vi "IMUOrientOpen.vi"(4 "Flash Drive?":bool, 5 "Stored Cal File":string="BNO055 Cal MC P3 11-28-2015 145653", 6 "Alt Adr":bool, 7 "Calibrate?":bool, 8 "Status delay":i32=30, 9 "I2C Bus":T2=enum."I2C MXP", 10 "Placement":T7(ring)=enum."P3", 11 "Op Mode":T5(ring)=enum."NDOF") -> (0 "Bad result":bool, 1 "Fatal Result":bool, 2 "Cal Status":T3, 3 "I2CDevRef":T1={"DevStatus"={"status"=FALSE, "code"=0, "source"=""}, "Device Address"=0, "Handle"=0, "I2C Bus"=enum."Invalid"} {"Device Address" format="%.0x"})   [LabVIEW 2015]
uses:
  <vilib>/Rock Robotics/SystemInterfaces/i2clib/i2c_bus.ctl
  Setup State.ctl
  <vilib>/Rock Robotics/WPI/I2C/WPI_I2CDevRef.ctl
panel:
  out "Adr":u8 format="%02x"
  out "Fatal Result":bool
  out "Restore Cal Ct":i32
  out "Bad ct":i32
  out "SC ct":i32
  out "S":T4
  out "G":T4
  out "A":T4
  out "M":T4
  out "Bad result":bool
  out "Fusion":bool
  out "Fusion ct":i32
  out "Reset ct":i32
  out "Occupant":u8[](array[numeric]) format="%02x"
  out "Setup ct":i32
  out "Setup State":T6
  # "Manual Cal\nCalibration Status Indicator"
  # "Diagnostics"
  # "These controls/indicators are non-operational / they are here as example documentation only."
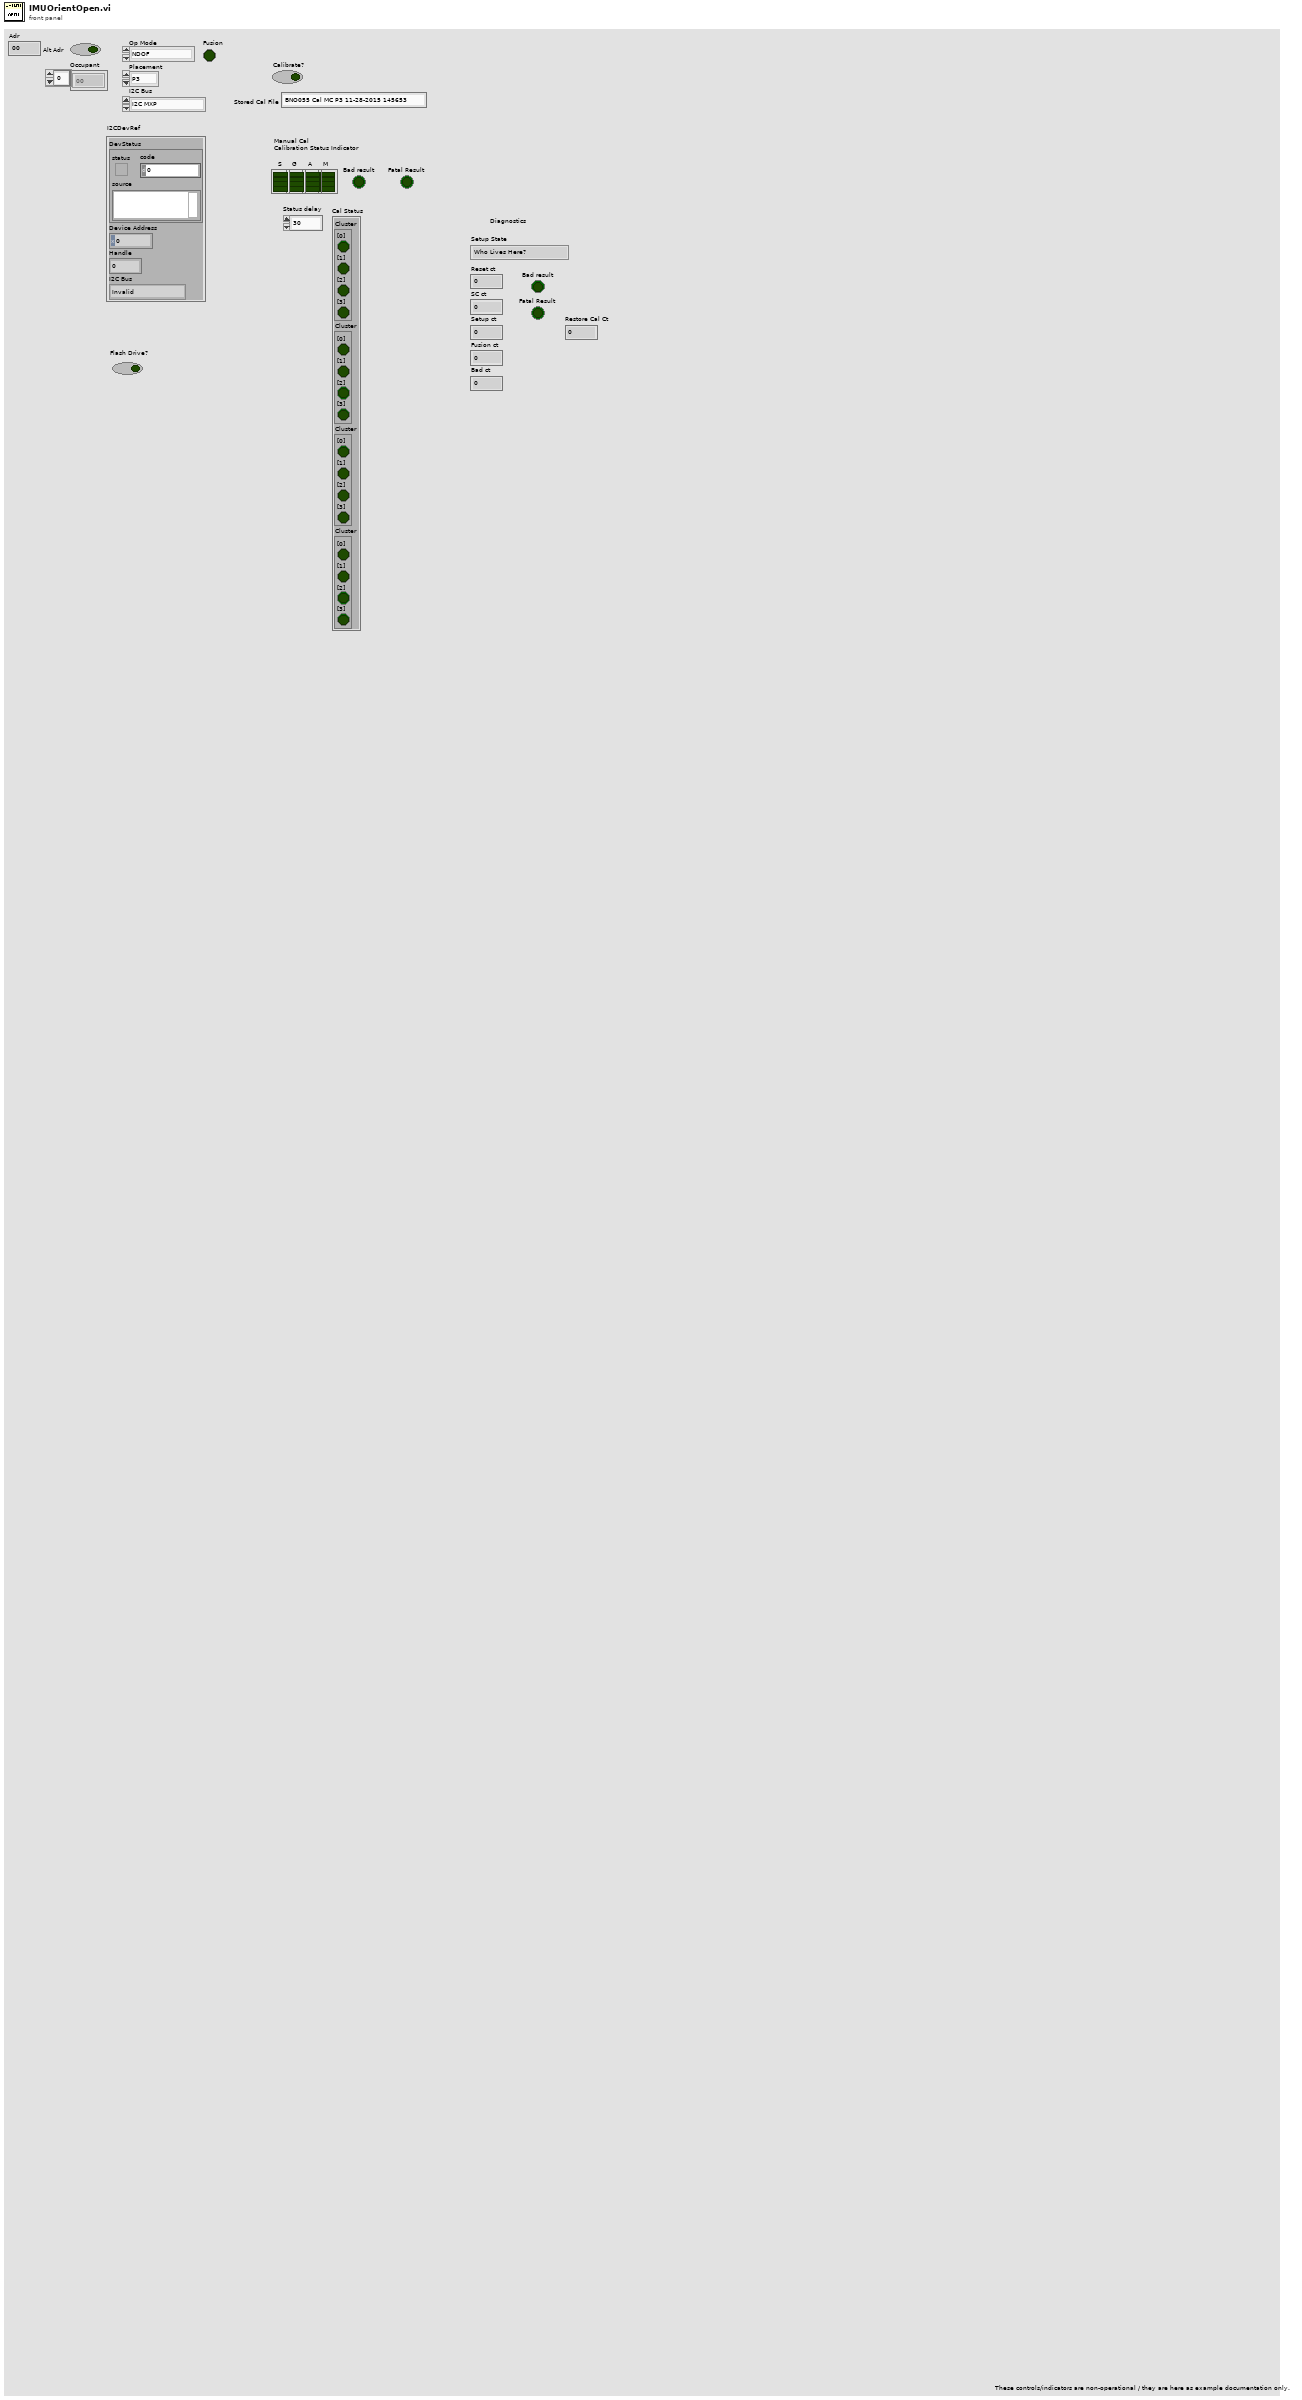
[diagram p1: front panel]
types:
  T1 = typedef "WPI_I2CDevRef.ctl" = cluster{"DevStatus":errorcluster, "Device Address":u8, "Handle":i32, "I2C Bus":T2}
  T2 = typedef "i2c_bus.ctl" = enum16{"I2C On-Board", "I2C MXP", "Invalid"}
  T3 = cluster{"Cluster":cluster{"[0]":bool, "[1]":bool, "[2]":bool, "[3]":bool}, "Cluster":cluster{"[0]":bool, "[1]":bool, "[2]":bool, "[3]":bool}, "Cluster":cluster{"[0]":bool, "[1]":bool, "[2]":bool, "[3]":bool}, "Cluster":cluster{"[0]":bool, "[1]":bool, "[2]":bool, "[3]":bool}}
  T4 = cluster{"Boolean":bool, "Boolean 2":bool, "Boolean 3":bool, "Boolean 4":bool}
  T5 = enum8{"ConfigMode", "AccOnly", "MagOnly", "GyroOnly", "AccMag", "AccGyro", "MagGyro", "AMG", "IMU", "Compass", "M4G", "NDOF_FMC_OFF", "NDOF"}
  T6 = typedef "Setup State.ctl" = enum16{"Who Lives Here?", "Config Mode", "Page 0", "Reset", "Units, Xtal, & Placement", "Fusion Mode", "Pre Calibration", "Error Check", "Manual Cal", "Save Cal", "Restore Cal", "Cal Status", "Idle"}
  T7 = enum32{"P0", "P1", "P2", "P3", "P4", "P5", "P6", "P7"}
  T8 = enum16{"open", "open or create", "create or replace", "create", "open (read-only)"}
  T9 = enum8{"ConfigMode", "AccOnly", "MagOnly", "GyroOnly", "AccMag", "AccGyro", "MagGyro", "AMG", "IMU", "Compass", "M4G", "NDOF_FMC_OFF", "NDOF"}[]
  T10 = cluster{"[0]":bool, "[1]":bool, "[2]":bool, "[3]":bool}
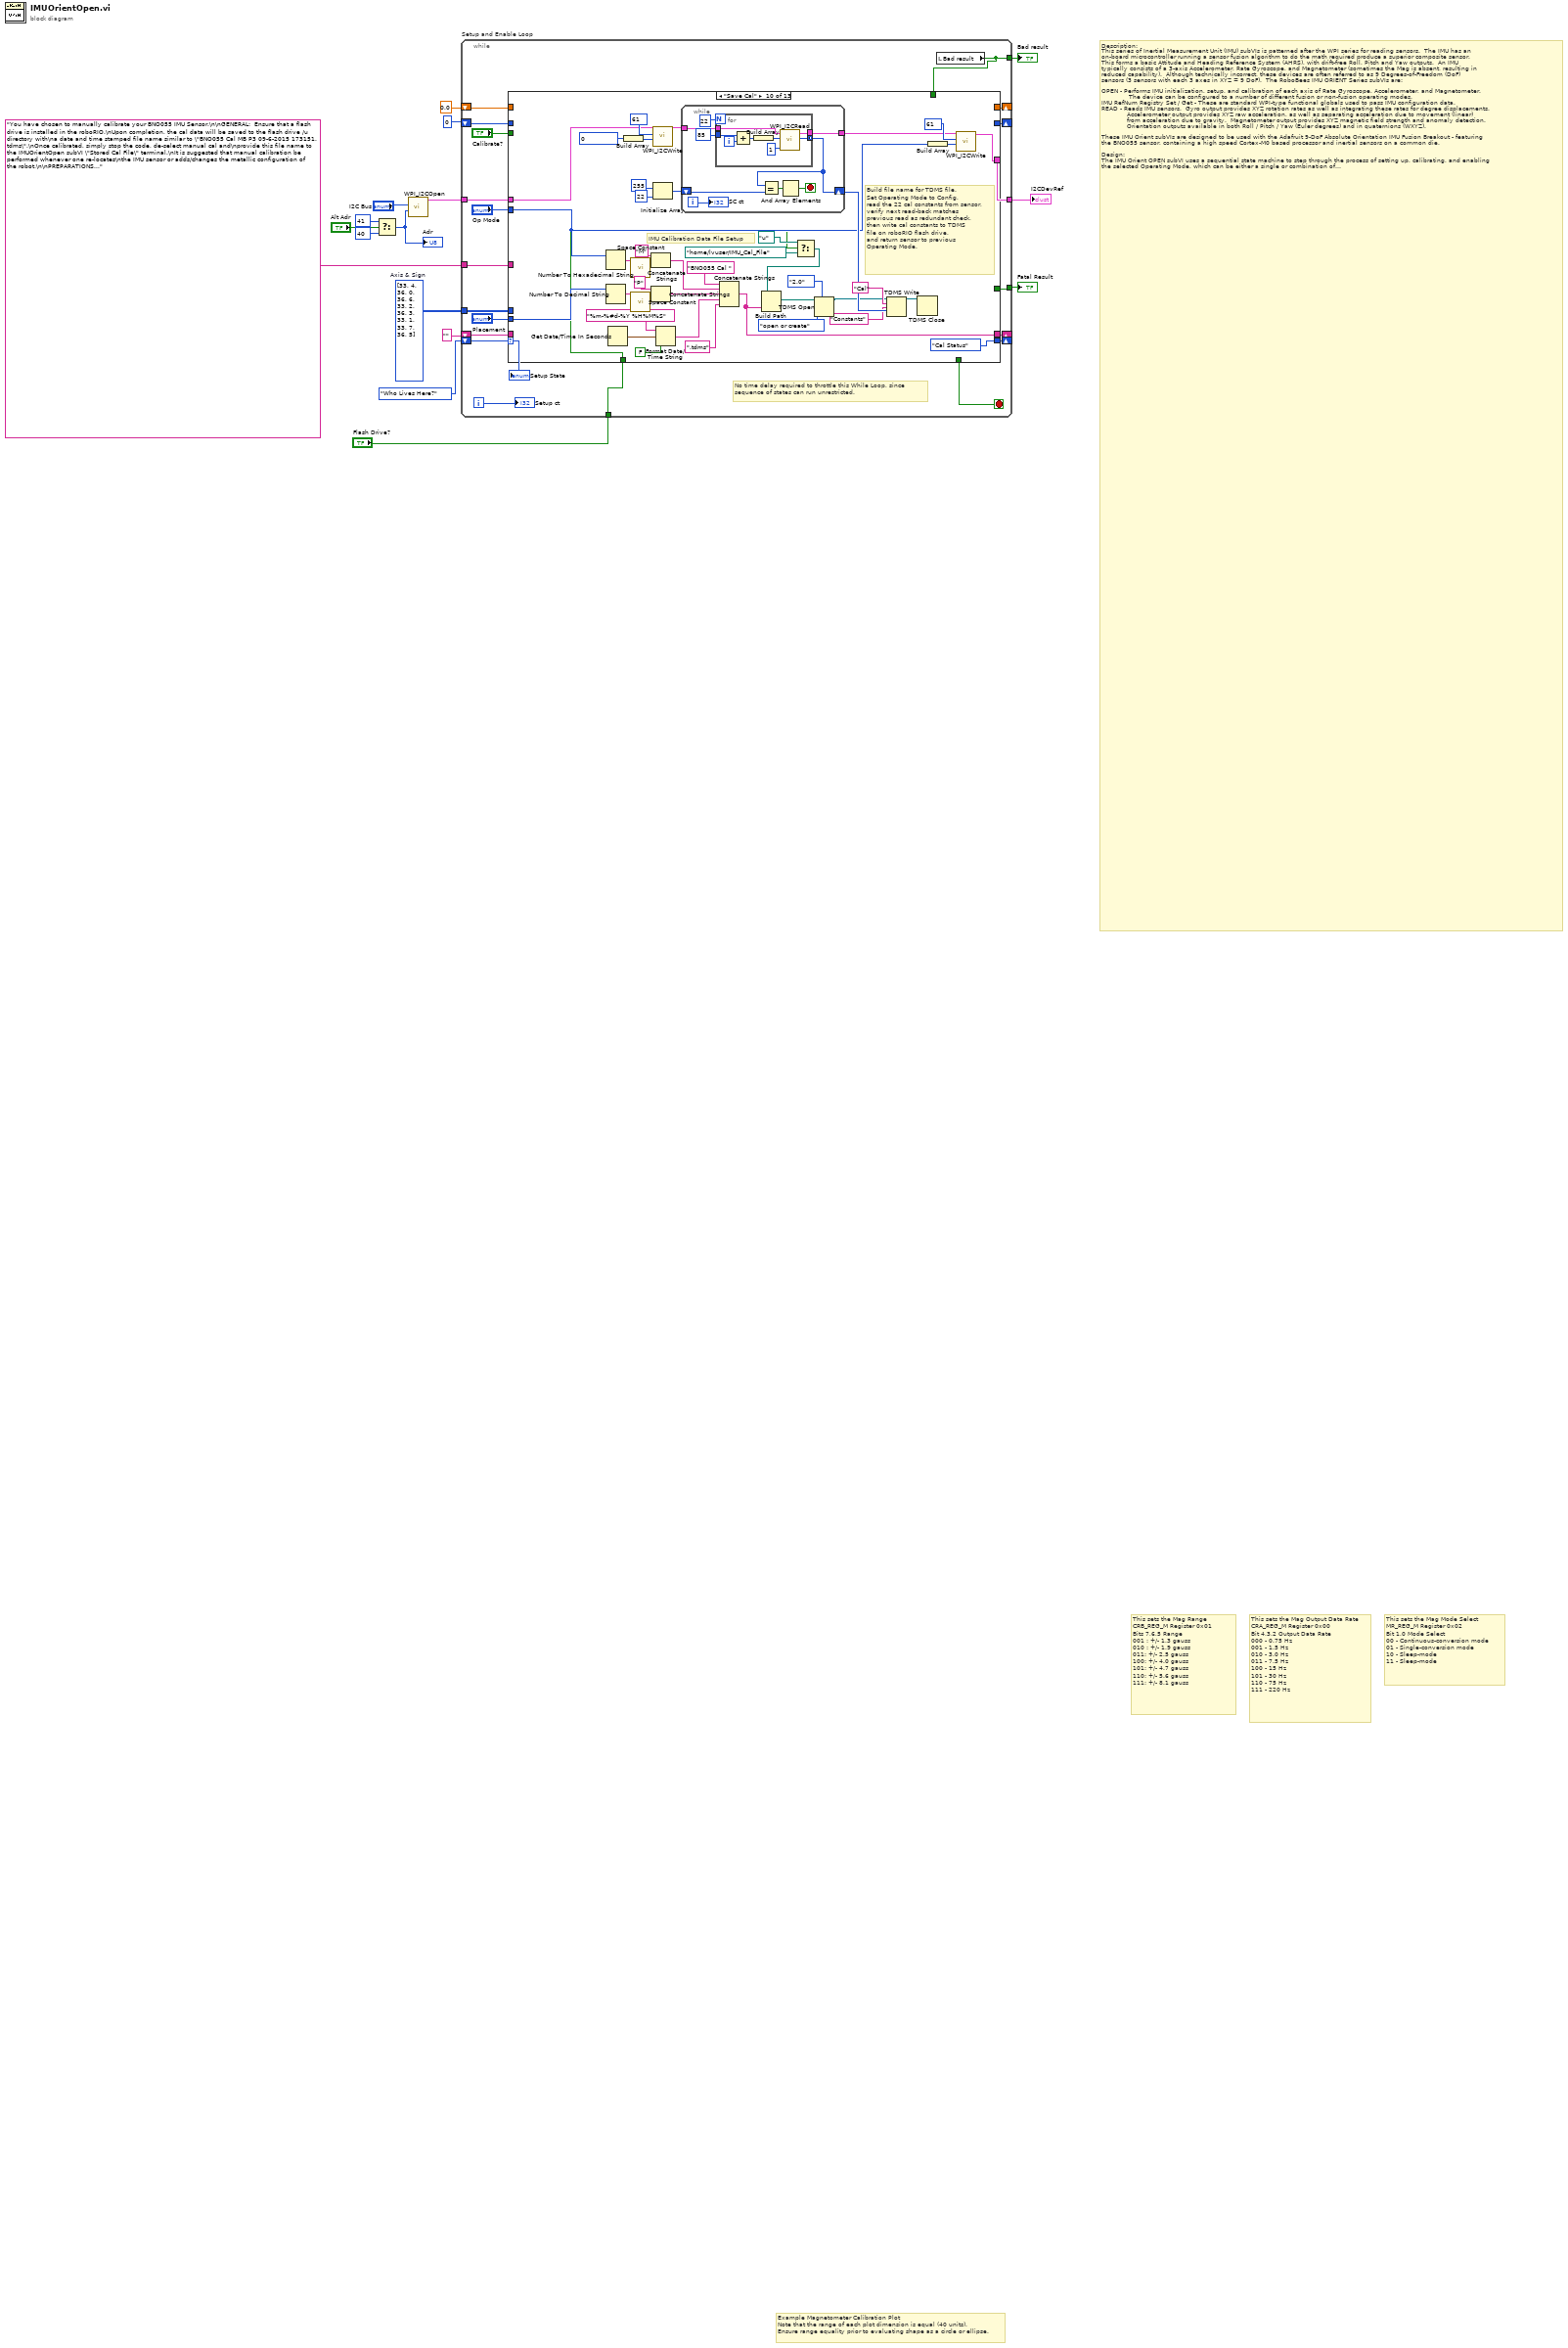
[diagram p0: block diagram]
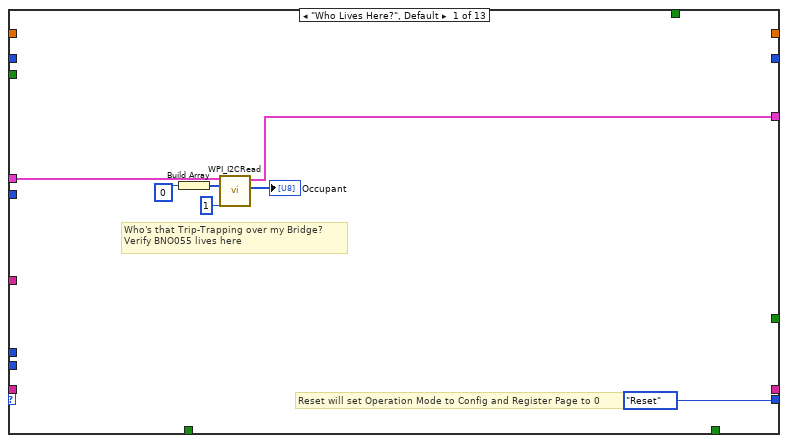
[diagram p2: hidden frame]
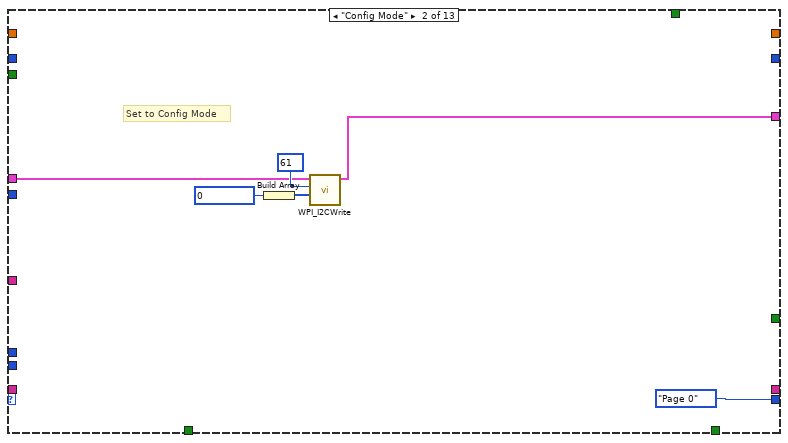
[diagram p3: hidden frame]
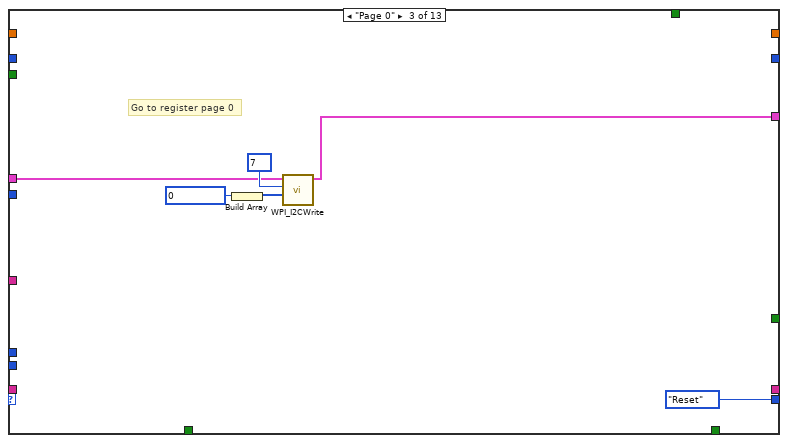
[diagram p4: hidden frame]
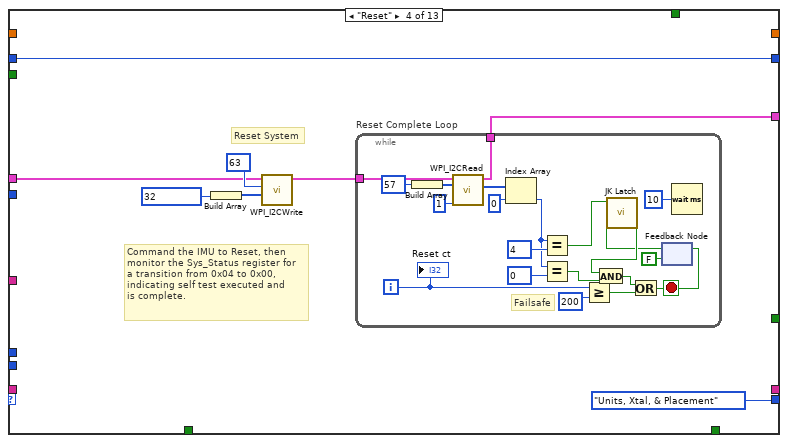
[diagram p5: hidden frame]
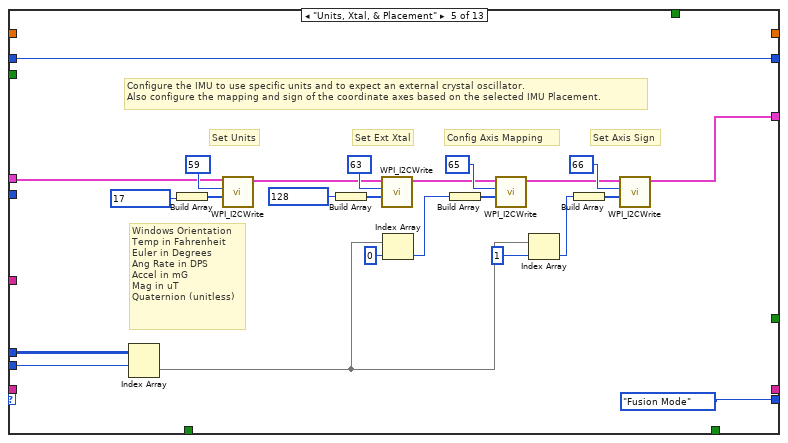
[diagram p6: hidden frame]
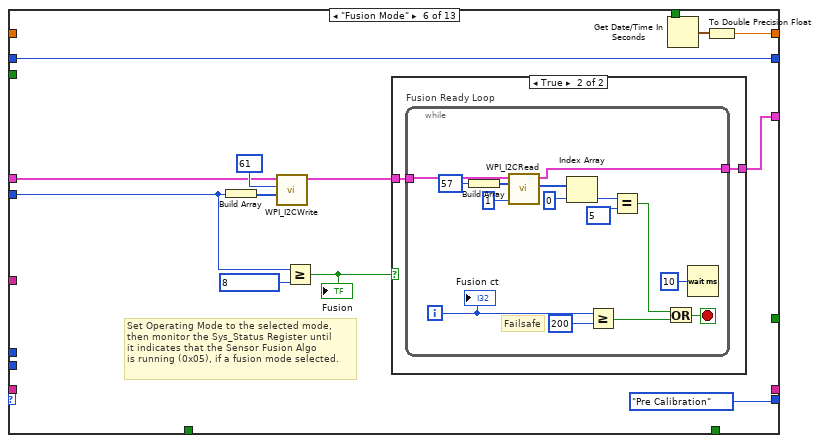
[diagram p7: hidden frame]
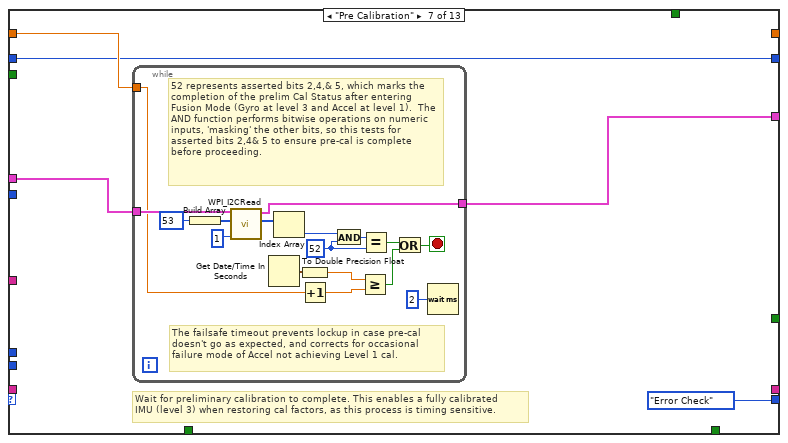
[diagram p9: hidden frame]
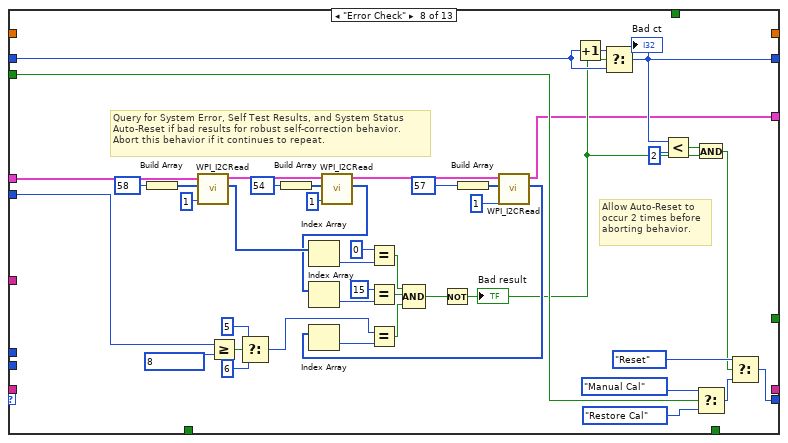
[diagram p10: hidden frame]
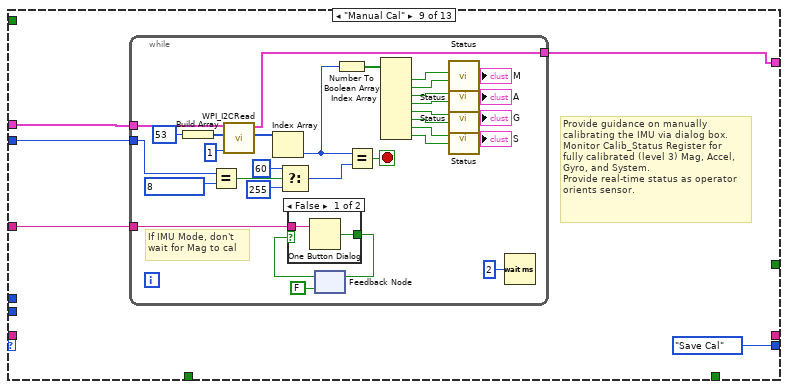
[diagram p11: hidden frame]
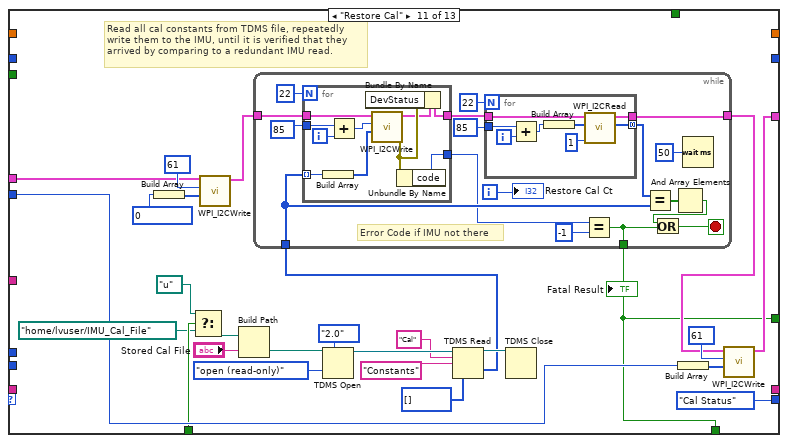
[diagram p13: hidden frame]
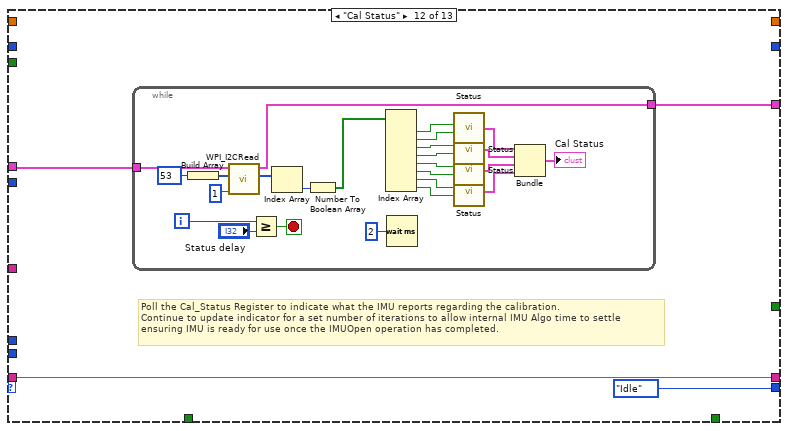
[diagram p14: hidden frame]
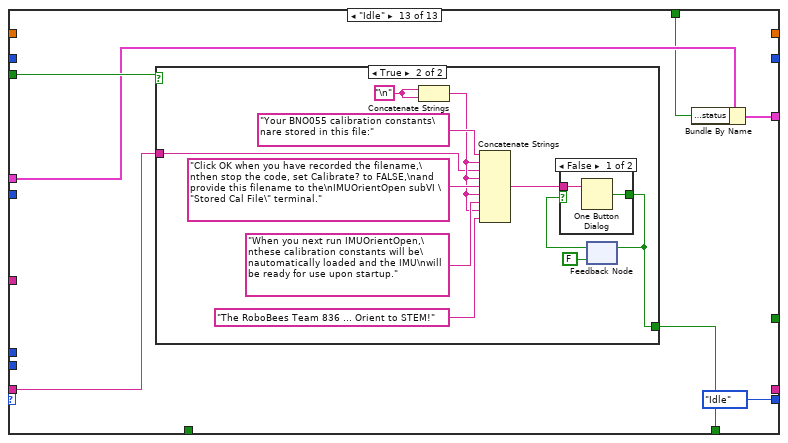
[diagram p15: hidden frame]
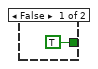
[diagram p16: hidden frame]
diagram:
  w13 = u8[][] [[33, 4], [36, 0], [36, 6], [33, 2], [36, 3], [33, 1], [33, 7], [36, 5]]  # Axis & Sign
  # "Description:\nThis series of Inertial Measurement Unit (IMU) subVIs is patterned after the WPI series for reading sensors.  The IMU has an\non-board microcontroller running a sensor fusion algorithm to do the math required produce a superior composite sensor.\nThis forms a basic Attitude and Heading Reference System (AHRS), with drift-free Roll, Pitch and Yaw outputs.  An IMU\ntypically consists of a 3-axis Accelerometer, Rate Gyroscope, and Magnetometer (sometimes the Mag is absent, resulting in\nreduced capability).  Although technically incorrect, these devices are often referred to as 9 Degrees-of-Freedom (DoF)\nsensors (3 sensors with each 3 axes in XYZ = 9 DoF).  The RoboBees IMU ORIENT Series subVIs are:\n\nOPEN - Performs IMU initialization, setup, and calibration of each axis of Rate Gyroscope, Accelerometer, and Magnetometer.\n              The device can be configured to a number of different fusion or non-fusion operating modes.\nIMU RefNum Registry Set / Get - These are standard WPI-type functional globals used to pass IMU configuration data.\nREAD - Reads IMU sensors.  Gyro output provides XYZ rotation rates as well as integrating these rates for degree displacements.\n             Accelerometer output provides XYZ raw acceleration, as well as separating acceleration due to movement (linear)\n             from acceleration due to gravity.  Magnetometer output provides XYZ magnetic field strength and anomaly detection.\n             Orientation outputs available in both Roll / Pitch / Yaw (Euler degrees) and in quaternions (WXYZ).\n\nThese IMU Orient subVIs are designed to be used with the Adafruit 9-DoF Absolute Orientation IMU Fusion Breakout - featuring\nthe BNO055 sensor, containing a high speed Cortex-M0 based processor and inertial sensors on a common die.\n\nDesign:\nThe IMU Orient OPEN subVI uses a sequential state machine to step through the process of setting up, calibrating, and enabling\nthe selected Operating Mode, which can be either a single or combination of sensors running in a non-fusion mode, or one of\nseveral fusion operating modes.\n\nThe IMU breakout board from Adafruit.com has a single I2C bus for communication.  The sensor I2C Address (in hex) and\nrespective data sheets for I2C register references are:\n\nI2C Address  -  Data Sheet Reference\n       0x28        -  http://ae-bst.resource.bosch.com/media/_tech/media/datasheets/BST_BNO055_DS000_13.pdf\n\nNote: The Adafruit website links to an older version of the BNO055 spec sheet (ver 1.2).  The Bosch site will maintain the latest\nversion.  The link above is the latest revision (ver 1.3) as of January 2016 (released August 2015).   This is a highly sophisticated\nsensor, with many control options, so it is recommended that one review the spec sheet to understand all its capabilities.\n\nSome design effort was expended in an attempt to ensure high reliability of operation.  Data transfer between the sensor cal registers\nand the required flash drive (where cal constants are stored during power down periods) is redundantly verified to be successful.  (Testing\nindicated this to be necessary.)  Upon initialization, if the sensor fails its internal self test, the code will attempt to reset the sensor.\nThis will only occur two times to avoid an infinite loop, which might otherwise prevent a robot from executing operations code.\n\nCalibration:\nRaw readings from an IMU are not very useful until they are conditioned by carefully determined calibration parameters.  One of\nthe key differences between this IMU and others, such as the one discussed here: \n\n                                                         http://www.chiefdelphi.com/forums/showthread.php?t=131823 \n\nis that this BNO055 contains an integrated microcontroller, running a sensor fusion algorithm, which is designed to constantly\nself-calibrate in real-time, after an initial calibration process has occurred.  So, unlike other IMUs that require interface code, this\nIMU really only requires code to trigger the on-board calibration code.  This makes the code for the sensor READ operations simple,\nand the complex code integration requirement associated only with the sensor OPEN (although one only has to trigger the on-board\ncal process, doing this reliably and providing functionality to store/reload the results still drives code sophistication requirements).\n\nOnce the state machine has initialized the sensor, a user-selected control is referenced to either initiate the sensor's embedded\ncal process or read previously stored calibration constants from a file.  [Note: this vi expects a flash drive to be installed in one\nof the roboRIOs USB ports for cal file storage/retrieval].   A dialog box is used to instruct the user on the sensor movements required\nfor calibration, and a Calibration Status Indicator is provided on this vi's front panel to provide feedback and track progress.   Once\ncal is complete, the filename containing the cal constants is displayed.  De-selecting the cal control and providing the cal filename\nto this vi enables the sensor to open in a ready-for-use state.\n\nThe cal filename will contain the Operating Mode, Placement (sensor orientation), and a timestamp to help distinguish one file\nfrom another.  The Op Mode and Placement are included as there is some indication in testing that one should not expect the cal\nto be correct when these parameters differ between cal and use.\n\nVI Properties:\nExecution Reentrancy is set to Non Reentrant Execution\n\nImplementation:\nIt is recommended that the MXP I2C Interface is used, rather than the On-Board I2C Interface, as the latter can generate glitches from\nLo/Hi byte pairing failures when data is reassembled across paired measurement registers.\n\nA visualization vi is provided to observe orientation change as the sensor is moved.  The vi runs on the My Computer Target,\n(not the roboRIO Target), which means it can only be accessed in debug mode.  There is an issue where Roll exceeding ~45 degrees\ncauses an orientation error.\n \nIt is important to note that while the P/R/Y values are constrained, the Gyro displacement values in X/Y/Z are not.  Gyro deg outputs\nfrom the IMU ORIENT READ subVI will wind (not wrap) - i.e. they will continue to count above/below 360 degrees.  Use the LabVIEW\nQuotient & Remainder (modulus) function to convert these outputs to a wrapping behavior, if desired. \n\nImplementation considerations for IMU Read:\nThis design performs numerical integration off-FPGA for the Digital Gyro (unlike the Analog Gyro subVIs, which typically utilize\nthe FPGA to perform accumulation for superior speed resulting in less integration error).   Testing indicates this off-FPGA\napproach may be adequate for FRC application, however, it is important to ensure the code runs without any timing issues.\nThis is why a Timed Loop is recommended for the IMU Read within Periodic Tasks (executes at a higher priority).  Non-uniformity\nin read iteration is mitigated by design, as each dt is uniquely calculated by time stamping each read event.  This means that while\nsome variation in timing can be tolerated (the occasional late iteration), excessively long durations (periods) between successive\nreads will fail to capture the actual rate profile as it changes resulting in integration error.  \n\nIn short, use a Timed Loop structure to iterate IMU READs, and set the loop period for a relatively fast iteration (<75 ms).  Shorter\nperiods provide improved accuracy of degree displacements, however setting this too short can impact the execution of your\nremaining code (especially when using Timed Loops).  One way of determining an optimized period is to set it while monitoring\nthe \"Finished Late?\" Loop parameter, ensuring this value stays False.   It helps if the CPU Utilization remains low (<75%), which\ncan be monitored with the RT Get CPU Loads subVI (Real Time menu).  Study LabVIEW determinism for additional insight.\n\n----- RoboBees FRC Team 836! -----  You too can conquer inertia!! ... ORIENT on a career in STEM!"
  # "Example Magnetometer Calibration Plot\nNote that the range of each plot dimension is equal (40 units).\nEnsure range equality prior to evaluating shape as a circle or ellipse."
  # "This sets the Mag Mode Select\nMR_REG_M Register 0x02\nBit 1,0 Mode Select\n00 - Continuous-conversion mode \n01 - Single-conversion mode\n10 - Sleep-mode\n11 - Sleep-mode"
  # "This sets the Mag Output Data Rate\nCRA_REG_M Register 0x00\nBit 4,3,2 Output Data Rate\n000 - 0.75 Hz \n001 - 1.5 Hz \n010 - 3.0 Hz\n011 - 7.5 Hz\n100 - 15 Hz\n101 - 30 Hz\n110 - 75 Hz\n111 - 220 Hz"
  # "This sets the Mag Range\nCRB_REG_M Register 0x01\nBits 7,6,5 Range\n001 : +/- 1.3 gauss\n010 : +/- 1.9 gauss\n011: +/- 2.5 gauss\n100: +/- 4.0 gauss\n101: +/- 4.7 gauss\n110: +/- 5.6 gauss\n111: +/- 8.1 gauss"
  n1 = Select(t=u8 41 ("Device Address"), s="Alt Adr", f=u8 40 ("Device Address")) -> (s? t:f=w3:u8)
  "Adr" <- w3
  n2 = call <vilib>:"WPI_I2COpen.vi"("Device Address"=w3, "I2C Bus"="I2C Bus") -> ("I2CDevRef"=w14:T1)  [unwired: 8 in, 1 out]
  n3 = while "Setup and Enable Loop" {
    tunnel: w14 -> [w30]
    tunnel: "You have chosen to manually calibrate your BNO055 IMU Sensor.\n\nGENERAL:  Ensure that a flash drive is installed in the roboRIO.\nUpon completion, the cal data will be saved to the flash drive /u directory with\na date and time stamped file name similar to \"BNO055 Cal MB P3 09-6-2015 173151.tdms\".\nOnce calibrated, simply stop the code, de-select manual cal and\nprovide this file name to the IMUOrientOpen subVI \"Stored Cal File\" terminal.\nIt is suggested that manual calibration be performed whenever one re-locates\nthe IMU sensor or adds/changes the metallic configuration of the robot.\n\nPREPARATIONS:  If sensor is installed on a robot, ensure sensor is secure.\nThese device movement instructions will then apply to entire robot.\nAs you proceed, monitor the Calibration Status Indicator on the IMUOrientOpen Front Panel.\nCalibration is complete when all indicators are Green.\n\nGYRO CAL:  Allow device to maintain a single stable\nposition to enable Gyro to self-calibrate.\n\nACCELEROMETER CAL:  Place device in 6 different stable\npositions for a few seconds to allow it to calibrate.\nEnsure there is slow movement between 2 stable positions.\nThe 6 stable positions can be in any direction, but ensure the\ndevice is perpendicular to the X,Y & Z axis at least once.\nThis is usually the most difficult device to calibrate.\nIf problematic, try slowing down the movement between positions.\n\nMAGNETOMETER CAL:  Make random movements\nin all 3 axes until Cal Status Indicator is Green.\n\nSYSTEM CAL:  Alternately move device and hold still until\nCal Status Indicator is Green, if necessary. \n\nClick OK when ready to begin." ("message") -> [w35]
    tunnel: w13 -> [w33]
    tunnel: [w19] -> w12
    shift-right: [w28] -> _
    shift-left: 0 -> [w27]
    tunnel: [w18] -> w10
    shift-right: [w26] -> _
    shift-left: 0.0 -> [w25]
    shift-right: [w24] -> _
    shift-left: "" -> [w23]
    shift-right: [w22] -> _
    shift-left: Setup_State."Who Lives Here?" -> [w21]
    tunnel: [w20] -> w6
    tunnel: "Flash Drive?" -> [w17]
    i -> [w32]
    stop <- w31 stop-if-true
    # "No time delay required to throttle this While Loop, since sequence of states can run unrestricted."
    n4 = local read "Bad result"() -> (w18:bool)
    n5 = case shown="\"Save Cal\"" w21 {
      tunnel: [Setup_State."Reset" Setup_State."Page 0" Setup_State."Reset" Setup_State."Units, Xtal, & Placement" Setup_State."Fusion Mode" Setup_State."Pre Calibration" Setup_State."Error Check" w177 Setup_State."Save Cal" Setup_State."Cal Status" Setup_State."Cal Status" Setup_State."Idle" Setup_State."Idle"] -> w22
      tunnel: w30 -> [w40 w45 w52 w60 w100 w118 w143 w193 w209 w280 w316 w368 w396]
      tunnel: "Calibrate?" -> [_ _ _ _ _ _ _ w165 _ _ _ _ w400]
      tunnel: [_ _ _ _ _ w115 _ _ _ _ _ _ _] -> w26
      tunnel: w25 -> [_ _ _ _ _ _ w141 _ _ _ _ _ _]
      tunnel: w35 -> [_ _ _ _ _ _ _ _ w207 _ _ _ _]
      tunnel: "Placement" -> [_ _ _ _ w90 _ _ _ _ w254 _ _ _]
      tunnel: w33 -> [_ _ _ _ w88 _ _ _ _ _ _ _ _]
      tunnel: [_ _ _ _ _ _ _ _ _ w251 _ w366 _] -> w24
      tunnel: [_ _ _ _ _ _ _ _ _ _ w308 _ w399] -> w31
      tunnel: w23 -> [_ _ _ _ _ _ _ _ _ _ _ w366 w398]
      tunnel: "Op Mode" -> [_ _ _ _ _ w111 _ w170 w205 w250 w311 _ _]
      tunnel: [_ _ _ w57 w86 w110 w140 w167 _ _ _ _ _] -> w28
      tunnel: w27 -> [_ _ _ w57 w86 w110 w140 w168 _ _ _ _ _]
      tunnel: [_ _ _ _ _ _ _ _ _ _ w308 _ _] -> w20
      tunnel: [w37 w44 w50 w56 w85 w109 w139 w161 w206 w249 w309 w365 w395] -> w19
      tunnel: w18 -> [_ _ _ _ _ _ _ _ _ _ _ _ w394]
      tunnel: w17 -> [_ _ _ _ _ _ _ _ _ w245 w307 _ _]
      frame "Who Lives Here?", Default {
        # "Reset will set Operation Mode to Config and Register Page to 0"
        # "Who's that Trip-Trapping over my Bridge?\nVerify BNO055 lives here"
        n6 = Build Array(u8 0 ("Data To Send")) -> (w43:u8[])
        n7 = call <vilib>:"WPI_I2CRead.vi"("I2CBytesToRead"=u8 1, "I2CRegister"=w43, "I2CDevRef"=w40) -> ("Data Out"=→"Occupant":u8[], "I2CDevRef"=w37:T1)  [unwired: 6 in, 1 out]
      }
      frame "Config Mode" {
        # "Set to Config Mode"
        n8 = Build Array(u8 0 ("I2CRegister")) -> (w49:u8[])
        n9 = call <vilib>:"WPI_I2CWrite.vi"("I2CDataToSend"=w49, "I2CRegister"=u8 61 ("Data To Send hex 2"), "I2CDevRef"=w45) -> ("I2CDevRef"=w44:T1)  [unwired: 7 in, 1 out]
      }
      frame "Page 0" {
        # "Go to register page 0"
        n10 = Build Array(u8 0 ("I2CRegister")) -> (w55:u8[])
        n11 = call <vilib>:"WPI_I2CWrite.vi"("I2CDataToSend"=w55, "I2CRegister"=u8 7 ("Data To Send hex 2"), "I2CDevRef"=w52) -> ("I2CDevRef"=w50:T1)  [unwired: 7 in, 1 out]
      }
      frame "Reset" {
        # "Command the IMU to Reset, then\nmonitor the Sys_Status register for\na transition from 0x04 to 0x00,\nindicating self test executed and\nis complete."
        # "Reset System"
        n12 = Build Array(u8 32 ("I2CRegister")) -> (w63:u8[])
        n13 = call <vilib>:"WPI_I2CWrite.vi"("I2CDataToSend"=w63, "I2CRegister"=u8 63 ("Data To Send hex 2"), "I2CDevRef"=w60) -> ("I2CDevRef"=w58:T1)  [unwired: 7 in, 1 out]
        n14 = while "Reset Complete Loop" {
          tunnel: w58 -> [w79]
          tunnel: [w64] -> w56
          i -> [w67]
          stop <- w69 stop-if-true
          # "Failsafe"
          n15 = Build Array(u8 57 ("Data To Send")) -> (w82:u8[])
          n16 = call <vilib>:"WPI_I2CRead.vi"("I2CBytesToRead"=u8 1, "I2CRegister"=w82, "I2CDevRef"=w79) -> ("Data Out"=w81:u8[], "I2CDevRef"=w64:T1)  [unwired: 6 in, 1 out]
          n17 = Index Array(array=w81, index=0 ("disabled index (col)")) -> (element=w68:u8)
          n18 = Equal?(x=w68, y=u8 4 ("I2CBytesToRead")) -> (x = y?=w74:bool)
          n19 = Equal?(x=w68, y=u8 0 ("I2CBytesToRead")) -> (x = y?=w73:bool)
          n20 = Greater Or Equal?(x=w67, y=200) -> (x >= y?=w71:bool)
          n21 = feedback #1(FALSE) -> (w66:bool)
          n22 = call "JK Latch.vi"("Reset"=w66, "Set"=w74) -> ("Q"=w75:bool)  [unwired: 5 in]
          n23 = And(x=w75, y=w73) -> (x .and. y?=w72:bool)
          n24 = Or(x=w72, y=w71) -> (x .or. y?=w69:bool)
          n25 = feedback-in #1(w69) -> ()
          n26 = Wait (ms)(milliseconds to wait=u32 10) -> ()  [unwired: 1 out]
          "Reset ct" <- w67
        }
      }
      frame "Units, Xtal, & Placement" {
        # "Configure the IMU to use specific units and to expect an external crystal oscillator.\nAlso configure the mapping and sign of the coordinate axes based on the selected IMU Placement."
        # "Set Axis Sign"
        # "Config Axis Mapping"
        # "Set Ext Xtal"
        # "Windows Orientation\nTemp in Fahrenheit\nEuler in Degrees\nAng Rate in DPS\nAccel in mG\nMag in uT\nQuaternion (unitless)"
        # "Set Units"
        n27 = Index Array(array=w88, index (row)=w90) -> (element=w91:u8[])  [unwired: 1 in]
        n28 = Build Array(u8 17 ("I2CRegister")) -> (w108:u8[])
        n29 = call <vilib>:"WPI_I2CWrite.vi"("I2CDataToSend"=w108, "I2CRegister"=u8 59 ("Data To Send hex 2"), "I2CDevRef"=w100) -> ("I2CDevRef"=w102:T1)  [unwired: 7 in, 1 out]
        n30 = Build Array(u8 128 ("I2CRegister")) -> (w107:u8[])
        n31 = call <vilib>:"WPI_I2CWrite.vi"("I2CDataToSend"=w107, "I2CRegister"=u8 63 ("Data To Send hex 2"), "I2CDevRef"=w102) -> ("I2CDevRef"=w97:T1)  [unwired: 7 in, 1 out]
        n32 = Index Array(array=w91, index=0) -> (element=w89:u8)
        n33 = Build Array(w89) -> (w98:u8[])
        n34 = call <vilib>:"WPI_I2CWrite.vi"("I2CDataToSend"=w98, "I2CRegister"=u8 65 ("Data To Send hex 2"), "I2CDevRef"=w97) -> ("I2CDevRef"=w94:T1)  [unwired: 7 in, 1 out]
        n35 = Index Array(array=w91, index=1) -> (element=w87:u8)
        n36 = Build Array(w87) -> (w96:u8[])
        n37 = call <vilib>:"WPI_I2CWrite.vi"("I2CDataToSend"=w96, "I2CRegister"=u8 66 ("Data To Send hex 2"), "I2CDevRef"=w94) -> ("I2CDevRef"=w85:T1)  [unwired: 7 in, 1 out]
      }
      frame "Fusion Mode" {
        # "Set Operating Mode to the selected mode,\nthen monitor the Sys_Status Register until\nit indicates that the Sensor Fusion Algo\nis running (0x05), if a fusion mode selected."
        n38 = Build Array(w111) -> (w120:T9)
        n39 = call <vilib>:"WPI_I2CWrite.vi"("I2CDataToSend"=w120, "I2CRegister"=u8 61 ("Data To Send hex 2"), "I2CDevRef"=w118) -> ("I2CDevRef"=w117:T1)  [unwired: 7 in, 1 out]
        n40 = Greater Or Equal?(x=w111, y=u8 8 ("I2CRegister")) -> (x >= y?=w113:bool)
        "Fusion" <- w113
        n41 = case shown="True" w113 {
          tunnel: w117 -> [w121 w123]
          tunnel: [w121 w122] -> w109
          frame False {
          }
          frame True {
            n42 = while "Fusion Ready Loop" {
              tunnel: w123 -> [w133]
              tunnel: [w124] -> w122
              i -> [w128]
              stop <- w132 stop-if-true
              # "Failsafe"
              n43 = Build Array(u8 57 ("Data To Send")) -> (w136:u8[])
              n44 = call <vilib>:"WPI_I2CRead.vi"("I2CBytesToRead"=u8 1, "I2CRegister"=w136, "I2CDevRef"=w133) -> ("Data Out"=w135:u8[], "I2CDevRef"=w124:T1)  [unwired: 6 in, 1 out]
              n45 = Index Array(array=w135, index=0 ("disabled index (col)")) -> (element=w125:u8)
              n46 = Greater Or Equal?(x=w128, y=200) -> (x >= y?=w129:bool)
              n47 = Equal?(x=w125, y=u8 5 ("I2CBytesToRead")) -> (x = y?=w131:bool)
              n48 = Or(x=w131, y=w129) -> (x .or. y?=w132:bool)
              n49 = Wait (ms)(milliseconds to wait=u32 10) -> ()  [unwired: 1 out]
              "Fusion ct" <- w128
            }
          }
        }
        n50 = Get Date/Time In Seconds() -> (seconds since 1Jan1904=w116:timestamp)
        n51 = To Double Precision Float(number=w116) -> (double precision float=w115:dbl)
      }
      frame "Pre Calibration" {
        # "Wait for preliminary calibration to complete. This enables a fully calibrated\nIMU (level 3) when restoring cal factors, as this process is timing sensitive."
        n52 = while {
          tunnel: w143 -> [w156]
          tunnel: w141 -> [w146]
          tunnel: [w144] -> w139
          stop <- w151 stop-if-true
          w152 = u8 52 ("y")
          # "The failsafe timeout prevents lockup in case pre-cal\ndoesn't go as expected, and corrects for occasional\nfailure mode of Accel not achieving Level 1 cal."
          # "52 represents asserted bits 2,4,& 5, which marks the completion of the prelim Cal Status after entering Fusion Mode (Gyro at level 3 and Accel at level 1).  The AND function performs bitwise operations on numeric inputs, 'masking' the other bits, so this tests for asserted bits 2,4& 5 to ensure pre-cal is complete before proceeding."
          n53 = Build Array(u8 53 ("Data To Send")) -> (w160:u8[])
          n54 = call <vilib>:"WPI_I2CRead.vi"("I2CBytesToRead"=u8 1, "I2CRegister"=w160, "I2CDevRef"=w156) -> ("Data Out"=w157:u8[], "I2CDevRef"=w144:T1)  [unwired: 6 in, 1 out]
          n55 = Get Date/Time In Seconds() -> (seconds since 1Jan1904=w150:timestamp)
          n56 = Index Array(array=w157) -> (element=w153:u8)  [unwired: 1 in]
          n57 = To Double Precision Float(number=w150) -> (double precision float=w147:dbl)
          n58 = Increment(x=w146) -> (x+1=w145:dbl)
          n59 = And(x=w153, y=w152) -> (x .and. y?=w154:u8)
          n60 = Greater Or Equal?(x=w147, y=w145) -> (x >= y?=w148:bool)
          n61 = Equal?(x=w154, y=w152) -> (x = y?=w149:bool)
          n62 = Or(x=w149, y=w148) -> (x .or. y?=w151:bool)
          n63 = Wait (ms)(milliseconds to wait=u32 2 ("pre-cal wait")) -> ()  [unwired: 1 out]
        }
      }
      frame "Error Check" {
        # "Allow Auto-Reset to\noccur 2 times before\naborting behavior."
        # "Query for System Error, Self Test Results, and System Status\nAuto-Reset if bad results for robust self-correction behavior.\nAbort this behavior if it continues to repeat."
        n64 = Build Array(u8 58 ("Data To Send")) -> (w202:u8[])
        n65 = call <vilib>:"WPI_I2CRead.vi"("I2CBytesToRead"=u8 1, "I2CRegister"=w202, "I2CDevRef"=w193) -> ("Data Out"=w184:u8[], "I2CDevRef"=w195:T1)  [unwired: 6 in, 1 out]
        n66 = Greater Or Equal?(x=w170, y=u8 8 ("I2CRegister")) -> (x >= y?=w175:bool)
        n67 = Select(t=u8 5 ("x"), s=w175, f=u8 6 ("x")) -> (s? t:f=w172:u8)
        n68 = Build Array(u8 54 ("Data To Send")) -> (w201:u8[])
        n69 = Index Array(array=w184) -> (element=w185:u8)  [unwired: 1 in]
        n70 = call <vilib>:"WPI_I2CRead.vi"("I2CBytesToRead"=u8 1, "I2CRegister"=w201, "I2CDevRef"=w195) -> ("Data Out"=w183:u8[], "I2CDevRef"=w194:T1)  [unwired: 6 in, 1 out]
        n71 = Index Array(array=w183) -> (element=w186:u8)  [unwired: 1 in]
        n72 = Equal?(x=u8 0, y=w185) -> (x = y?=w189:bool)
        n73 = Equal?(x=u8 15, y=w186) -> (x = y?=w190:bool)
        n74 = Build Array(u8 57 ("Data To Send")) -> (w196:u8[])
        n75 = call <vilib>:"WPI_I2CRead.vi"("I2CBytesToRead"=u8 1, "I2CRegister"=w196, "I2CDevRef"=w194) -> ("Data Out"=w182:u8[], "I2CDevRef"=w161:T1)  [unwired: 6 in, 1 out]
        n76 = Index Array(array=w182) -> (element=w188:u8)  [unwired: 1 in]
        n77 = Equal?(x=w172, y=w188) -> (x = y?=w191:bool)
        n78 = Compound Arithmetic op=AND(w189, w190, w191) -> (w192:bool)
        n79 = Not(x=w192) -> (.not. x?=w163:bool)
        "Bad result" <- w163
        n80 = Increment(x=w168) -> (x+1=w169:i32)
        n81 = Select(t=w169, s=w163, f=w168) -> (s? t:f=w167:i32)
        "Bad ct" <- w167
        n82 = Less?(x=w167, y=2) -> (x < y?=w162:bool)
        n83 = And(x=w162, y=w163) -> (x .and. y?=w164:bool)
        n84 = Select(t=Setup_State."Manual Cal", s=w165, f=Setup_State."Restore Cal") -> (s? t:f=w178:T6)
        n85 = Select(t=Setup_State."Reset", s=w164, f=w178) -> (s? t:f=w177:T6)
      }
      frame "Manual Cal" {
        # "Provide guidance on manually\ncalibrating the IMU via dialog box.\nMonitor Calib_Status Register for\nfully calibrated (level 3) Mag, Accel,\nGyro, and System. \nProvide real-time status as operator\norients sensor."
        n86 = while {
          tunnel: w209 -> [w238]
          tunnel: w207 -> [w219]
          tunnel: [w217] -> w206
          tunnel: w205 -> [w215]
          stop <- w218 stop-if-true
          # "If IMU Mode, don't\nwait for Mag to cal"
          n87 = Build Array(u8 53 ("Data To Send")) -> (w241:u8[])
          n88 = Equal?(x=w215, y=u8 8 ("I2CRegister")) -> (x = y?=w211:bool)
          n89 = call <vilib>:"WPI_I2CRead.vi"("I2CBytesToRead"=u8 1, "I2CRegister"=w241, "I2CDevRef"=w238) -> ("Data Out"=w239:u8[], "I2CDevRef"=w217:T1)  [unwired: 6 in, 1 out]
          n90 = Index Array(array=w239) -> (element=w223:u8)  [unwired: 1 in]
          n91 = Select(t=u8 60 ("y"), s=w211, f=u8 255 ("y")) -> (s? t:f=w210:u8)
          n92 = feedback #2(FALSE ("true")) -> (w221:bool)
          n93 = case shown="False" w221 {
            selector: w221 -> [_ w244]
            tunnel: [w243 w244] -> w222
            tunnel: w219 -> [w242 _]
            frame False {
              n94 = One Button Dialog(message=w242) -> (true=w243:bool)  [unwired: 1 in]
            }
            frame True {
            }
          }
          n95 = feedback-in #2(w222) -> ()
          n96 = Number To Boolean Array(number=w223) -> (Boolean array=w224:bool[])
          n97 = Equal?(x=w223, y=w210) -> (x = y?=w218:bool)
          n98 = Index Array(array=w224) -> (element #1=w236:bool, element #2=w235:bool, element #3=w234:bool, element #4=w233:bool, element #5=w232:bool, element #6=w231:bool, element #7=w230:bool, element #8=w229:bool)  [unwired: 8 in]
          n99 = call "Status.vi"("Big"=w235, "Little"=w236) -> ("Cluster"=→"M":T10)  [unwired: 2 in]
          n100 = call "Status.vi"("Big"=w233, "Little"=w234) -> ("Cluster"=→"A":T10)  [unwired: 2 in]
          n101 = call "Status.vi"("Big"=w231, "Little"=w232) -> ("Cluster"=→"G":T10)  [unwired: 2 in]
          n102 = call "Status.vi"("Big"=w229, "Little"=w230) -> ("Cluster"=→"S":T10)  [unwired: 2 in]
          n103 = Wait (ms)(milliseconds to wait=u32 2 ("pre-cal wait")) -> ()  [unwired: 1 out]
        }
      }
      frame "Save Cal" {
        # "Build file name for TDMS file.\nSet Operating Mode to Config,\nread the 22 cal constants from sensor,\nverify next read-back matches\nprevious read as redundant check,\nthen write cal constants to TDMS\nfile on roboRIO flash drive,\nand return sensor to previous\nOperating Mode."
        # "IMU Calibration Data File Setup"
        n104 = Number To Hexadecimal String(2:w250) -> (0:w257:string)  [unwired: 1 in]
        n105 = Number To Decimal String(number=w254) -> (decimal integer string=w261:string)  [unwired: 1 in]
        n106 = Get Date/Time In Seconds() -> (seconds since 1Jan1904=w265:timestamp)
        n107 = Build Array(u8 0 ("I2CRegister")) -> (w284:u8[])
        n108 = call <vilib>:"Space Constant.vi"() -> ("String"=w259:string)
        n109 = call <vilib>:"Space Constant.vi"() -> ("String"=w260:string)
        n110 = Concatenate Strings("M" ("string"), w257, w259) -> (w256:string)
        n111 = Concatenate Strings("P" ("string"), w261, w260) -> (w255:string)
        n112 = call <vilib>:"WPI_I2CWrite.vi"("I2CDataToSend"=w284, "I2CRegister"=u8 61 ("Data To Send hex 2"), "I2CDevRef"=w280) -> ("I2CDevRef"=w279:T1)  [unwired: 7 in, 1 out]
        n113 = Initialize Array(u8 255, 22 ("dimension size")) -> (w272:u8[])
        n114 = Format Date/Time String(time format string (%c)="%m-%#d-%Y %H%M%S", seconds (now)=w265, UTC format=FALSE) -> (date/time string=w263:string)
        n115 = while {
          tunnel: w279 -> [w290]
          shift-right: [w287] -> w276
          shift-left: w272 -> [w293]
          tunnel: [w291] -> w277
          i -> [w289]
          stop <- w292 stop-if-true
          n116 = for {
            N: 22 -> [_]
            tunnel: u8 85 ("Data To Send 2") -> [w300]
            tunnel: [w298] -> w287 mode=concatenating
            tunnel: w290 -> [w297]
            tunnel: [w296] -> w291
            i -> [w299]
            n117 = Add(x=w300, y=w299) -> (x+y=w301:i32)
            n118 = Build Array(w301) -> (w302:i32[])
            n119 = call <vilib>:"WPI_I2CRead.vi"("I2CBytesToRead"=u8 1, "I2CRegister"=w302, "I2CDevRef"=w297) -> ("Data Out"=w298:u8[], "I2CDevRef"=w296:T1)  [unwired: 6 in, 1 out]
          }
          n120 = Equal?(x=w287, y=w293) -> (x = y?=w288:bool[])
          n121 = And Array Elements(Boolean array=w288) -> (logical AND=w292:bool)
          "SC ct" <- w289
        }
        n122 = Concatenate Strings("BNO055 Cal " ("string"), w256, w255, w263, ".tdms" ("string")) -> (w251:string)
        n123 = Select(t=path "u:/" ("file path (dialog if empty)"), s=w245, f=path "/home/lvuser/IMU_Cal_File" ("file path (dialog if empty)")) -> (s? t:f=w246:path)
        n124 = Build Path(base path=w246, name or relative path=w251) -> (appended path=w269:path)
        n125 = TDMS Open(7:enum16{"1.0", "2.0"}."2.0" ("file format version (2.0)"), 10:T8."open or create" ("operation (0:open)"), 11:w269) -> (3:w253:refnum<k34>)  [unwired: 4 in, 1 out]
        n126 = TDMS Write(0:w253, 5:"Cal" ("group name in (Untitled)"), 7:"Constants" ("channel name(s) in"), 9:w276) -> (4:w252:refnum<k34>)  [unwired: 2 in, 3 out]
        n127 = TDMS Close(11:w252) -> ()  [unwired: 1 in, 2 out]
        n128 = Build Array(w250) -> (w286:T9)
        n129 = call <vilib>:"WPI_I2CWrite.vi"("I2CDataToSend"=w286, "I2CRegister"=u8 61 ("Data To Send hex 2"), "I2CDevRef"=w277) -> ("I2CDevRef"=w249:T1)  [unwired: 7 in, 1 out]
      }
      frame "Restore Cal" {
        # "Read all cal constants from TDMS file, repeatedly\nwrite them to the IMU, until it is verified that they\narrived by comparing to a redundant IMU read."
        n130 = Build Array(u8 0 ("I2CRegister")) -> (w325:u8[])
        n131 = Select(t=path "u:/" ("file path (dialog if empty)"), s=w307, f=path "/home/lvuser/IMU_Cal_File" ("file path (dialog if empty)")) -> (s? t:f=w304:path)
        n132 = call <vilib>:"WPI_I2CWrite.vi"("I2CDataToSend"=w325, "I2CRegister"=u8 61 ("Data To Send hex 2"), "I2CDevRef"=w316) -> ("I2CDevRef"=w315:T1)  [unwired: 7 in, 1 out]
        n133 = Build Path(base path=w304, name or relative path="Stored Cal File") -> (appended path=w312:path)
        n134 = TDMS Open(7:enum16{"1.0", "2.0"}."2.0" ("file format version (2.0)"), 10:T8."open (read-only)" ("operation (0:open)"), 11:w312) -> (3:w323:refnum<k34>)  [unwired: 4 in, 1 out]
        n135 = TDMS Read(0:w323, 5:"Cal" ("group name in (Untitled)"), 7:"Constants" ("channel name(s) in"), 12:u8[] []) -> (4:w324:refnum<k34>, 10:w314:u8[])  [unwired: 4 in, 4 out]
        n136 = while {
          tunnel: w314 -> [w339]
          tunnel: w315 -> [w344]
          tunnel: [w338] -> w313
          tunnel: [w330] -> w308
          i -> [w335]
          stop <- w333 stop-if-true
          # "Error Code if IMU not there"
          n137 = for {
            N: 22 -> [_]
            tunnel: u8 85 ("Data To Send 2") -> [w362]
            tunnel: w339 -> [w360] mode=indexing
            tunnel: w344 -> [w361]
            tunnel: [w355] -> w341
            tunnel: [w358] -> w332
            i -> [w363]
            n138 = Build Array(w360) -> (w359:u8[])
            n139 = Add(x=w362, y=w363) -> (x+y=w364:i32)
            n140 = call <vilib>:"WPI_I2CWrite.vi"("I2CDataToSend"=w359, "I2CRegister"=w364, "I2CDevRef"=w361) -> ("error out"=w357:errorcluster, "I2CDevRef"=w356:T1)  [unwired: 7 in]
            n141 = Bundle By Name(cluster=w356, "DevStatus"=w357) -> (w355:T1)
            n142 = Unbundle By Name(w357) -> ("code"=w358:i32)
          }
          n143 = for {
            N: 22 -> [_]
            tunnel: u8 85 ("Data To Send 2") -> [w351]
            tunnel: [w350] -> w340 mode=concatenating
            tunnel: w341 -> [w349]
            tunnel: [w348] -> w338
            i -> [w347]
            n144 = Add(x=w351, y=w347) -> (x+y=w352:i32)
            n145 = Build Array(w352) -> (w353:i32[])
            n146 = call <vilib>:"WPI_I2CRead.vi"("I2CBytesToRead"=u8 1, "I2CRegister"=w353, "I2CDevRef"=w349) -> ("Data Out"=w350:u8[], "I2CDevRef"=w348:T1)  [unwired: 6 in, 1 out]
          }
          n147 = Equal?(x=w332, y=-1) -> (x = y?=w330:bool)
          n148 = Equal?(x=w340, y=w339) -> (x = y?=w337:bool[])
          n149 = And Array Elements(Boolean array=w337) -> (logical AND=w334:bool)
          n150 = Or(x=w334, y=w330) -> (x .or. y?=w333:bool)
          n151 = Wait (ms)(milliseconds to wait=u32 50) -> ()  [unwired: 1 out]
          "Restore Cal Ct" <- w335
        }
        n152 = TDMS Close(11:w324) -> ()  [unwired: 1 in, 2 out]
        n153 = Build Array(w311) -> (w329:T9)
        n154 = call <vilib>:"WPI_I2CWrite.vi"("I2CDataToSend"=w329, "I2CRegister"=u8 61 ("Data To Send hex 2"), "I2CDevRef"=w313) -> ("I2CDevRef"=w309:T1)  [unwired: 7 in, 1 out]
      }
      frame "Cal Status" {
        # "Poll the Cal_Status Register to indicate what the IMU reports regarding the calibration.\nContinue to update indicator for a set number of iterations to allow internal IMU Algo time to settle\nensuring IMU is ready for use once the IMUOpen operation has completed."
        n155 = while {
          tunnel: w368 -> [w380]
          tunnel: [w369] -> w365
          i -> [w379]
          stop <- w377 stop-if-true
          n156 = Build Array(u8 53 ("Data To Send")) -> (w381:u8[])
          n157 = call <vilib>:"WPI_I2CRead.vi"("I2CBytesToRead"=u8 1, "I2CRegister"=w381, "I2CDevRef"=w380) -> ("Data Out"=w392:u8[], "I2CDevRef"=w369:T1)  [unwired: 6 in, 1 out]
          n158 = Greater Or Equal?(x=w379, y="Status delay") -> (x >= y?=w377:bool)
          n159 = Index Array(array=w392) -> (element=w391:u8)  [unwired: 1 in]
          n160 = Number To Boolean Array(number=w391) -> (Boolean array=w390:bool[])
          n161 = Index Array(array=w390) -> (element #1=w384:bool, element #2=w385:bool, element #3=w371:bool, element #4=w393:bool, element #5=w386:bool, element #6=w387:bool, element #7=w388:bool, element #8=w389:bool)  [unwired: 8 in]
          n162 = Wait (ms)(milliseconds to wait=u32 2 ("pre-cal wait")) -> ()  [unwired: 1 out]
          n163 = call "Status.vi"("Big"=w385, "Little"=w384) -> ("Cluster"=w376:T10)  [unwired: 2 in]
          n164 = call "Status.vi"("Big"=w393, "Little"=w371) -> ("Cluster"=w375:T10)  [unwired: 2 in]
          n165 = call "Status.vi"("Big"=w387, "Little"=w386) -> ("Cluster"=w374:T10)  [unwired: 2 in]
          n166 = call "Status.vi"("Big"=w389, "Little"=w388) -> ("Cluster"=w373:T10)  [unwired: 2 in]
          n167 = Bundle("Cluster"=w376, "Cluster"=w375, "Cluster"=w374, "Cluster"=w373) -> (→"Cal Status":T3)  [unwired: 1 in]
        }
      }
      frame "Idle" {
        n168 = case shown="True" w400 {
          tunnel: [TRUE w405] -> w399
          tunnel: w398 -> [_ w402]
          frame False {
          }
          frame True {
            w408 = "\n"
            n169 = Concatenate Strings(w408, w408) -> (w404:string)
            n170 = Concatenate Strings("Your BNO055 calibration constants\nare stored in this file:" ("message"), w404, w402, w404, "Click OK when you have recorded the filename,\nthen stop the code, set Calibrate? to FALSE,\nand provide this filename to the\nIMUOrientOpen subVI \"Stored Cal File\" terminal." ("string"), w404, "When you next run IMUOrientOpen,\nthese calibration constants will be\nautomatically loaded and the IMU\nwill be ready for use upon startup." ("string"), w404, "The RoboBees Team 836 ... Orient to STEM!" ("string")) -> (w410:string)
            n171 = feedback #3(FALSE ("true")) -> (w412:bool)
            n172 = case shown="False" w412 {
              selector: w412 -> [_ w415]
              tunnel: [w414 w415] -> w405
              tunnel: w410 -> [w413 _]
              frame False {
                n173 = One Button Dialog(message=w413) -> (true=w414:bool)  [unwired: 1 in]
              }
              frame True {
              }
            }
            n174 = feedback-in #3(w405) -> ()
          }
        }
        n175 = Bundle By Name(cluster=w396, "DevStatus.status"=w394) -> (w395:T1)
      }
    }
    "Setup ct" <- w32
    "Setup State" <- w21
  }
  "I2CDevRef" <- w12
  "Bad result" <- w10
  "Fatal Result" <- w6
